vi "rise.vi"(11 "TF":bool) -> (3 "UP?":bool)   [LabVIEW 2017]
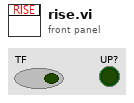
[diagram p1: front panel]
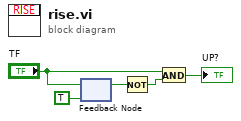
[diagram p0: block diagram]
diagram:
  n1 = feedback #1(TRUE ("B")) -> (w4:bool)
  n2 = feedback-in #1("TF") -> ()
  n3 = Not(x=w4) -> (.not. x?=w1:bool)
  n4 = And(x="TF", y=w1) -> (x .and. y?=→"UP?":bool)
